vi "Load Hardware.vi"(8 "error in (no error)":errorcluster, 10 "Program only changes":bool=TRUE, 11 "ArduinoDAC in":refnum<class "ArduinoDAC.lvclass">) -> (0 "error out":errorcluster, 3 "ArduinoDAC out":refnum<class "ArduinoDAC.lvclass">)   [LabVIEW 2013, in "ArduinoDAC.lvclass"]
uses:
  ArduinoDAC.lvclass
  <vilib>/Instr/_visa.llb/VISA Open Access Mode.ctl
  ArduinoDAC.lvclass/ArduinoDAC.ctl
panel:
  # "encapsulate HWI in cluser so each \"last encountered\"\ncan be a different length."
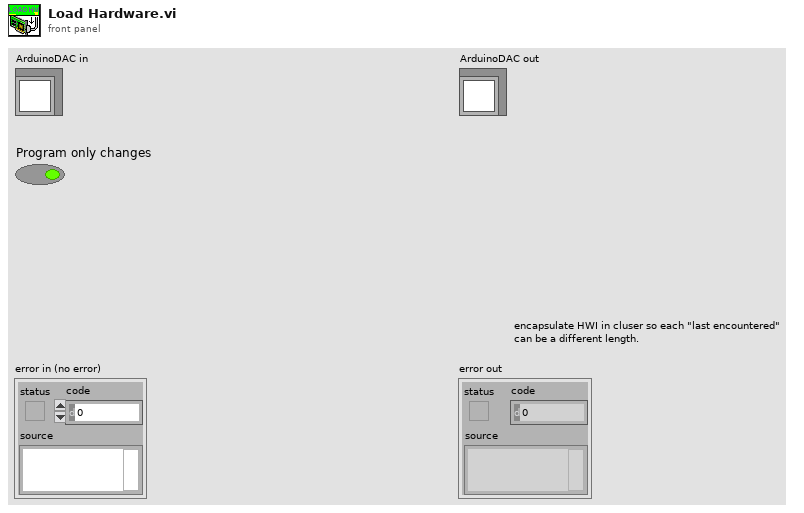
[diagram p1: front panel]
types:
  T1 = typedef "VISA Open Access Mode.ctl" = u32
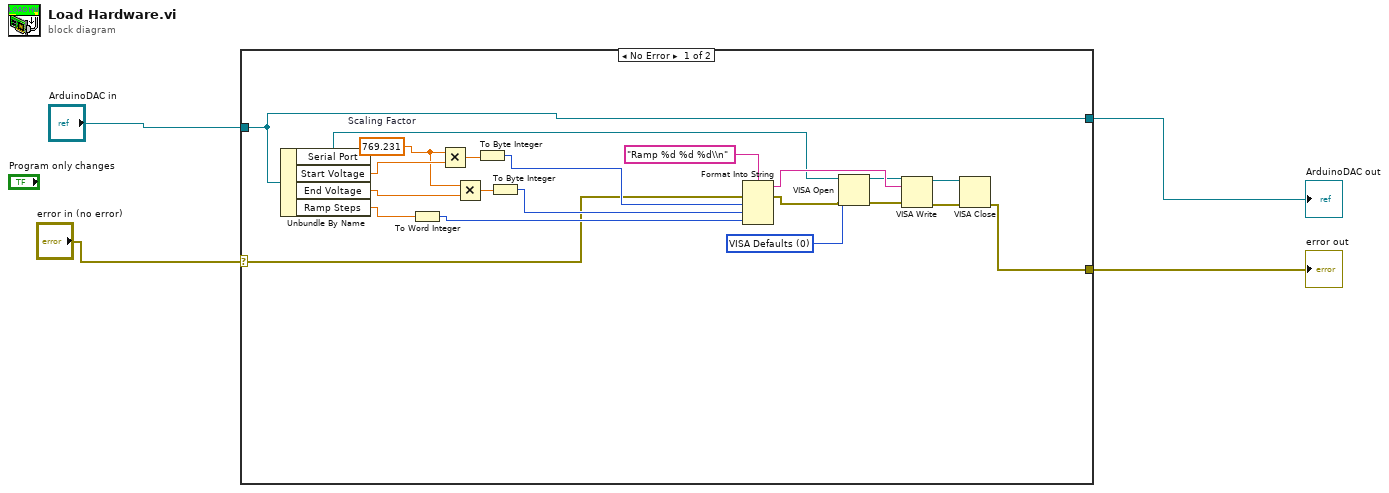
[diagram p0: block diagram]
diagram:
  n1 = case shown="No Error" "error in (no error)" {
    selector: "error in (no error)" -> [w14 w26]
    tunnel: "ArduinoDAC in" -> [w25 w27]
    tunnel: [w25 w27] -> w2
    tunnel: [w5 w26] -> w1
    frame No Error {
      w10 = T1 0 items=["VISA Defaults"=0, "Exclusive Lock"=1, "Load Configured Settings"=4] ("Access Mode")
      w23 = 769.231  # Scaling Factor
      n2 = Unbundle By Name(w25) -> ("Serial Port"=w12:refnum<visa-resource-name>, "Start Voltage"=w24:dbl, "End Voltage"=w22:dbl, "Ramp Steps"=w19:dbl)
      n3 = To Word Integer(number=w19) -> (16bit integer=w16:i16)
      n4 = Multiply(x=w23, y=w24) -> (x*y=w20:dbl)
      n5 = Multiply(x=w23, y=w22) -> (x*y=w21:dbl)
      n6 = To Byte Integer(number=w20) -> (8bit integer=w18:i8)
      n7 = To Byte Integer(number=w21) -> (8bit integer=w17:i8)
      n8 = Format Into String(format string="Ramp %d %d %d\\n", error in=w14, w18, w17, w16) -> (resulting string=w13:string, error out=w11:errorcluster)  [unwired: 1 in]
      n9 = VISA Open(access mode=w10, error in (no error)=w11, VISA resource name=w12) -> (VISA resource name=w9:refnum<visa-resource-name>, error out=w8:errorcluster)  [unwired: 2 in]
      n10 = VISA Write(VISA resource name=w9, write buffer=w13, error in (no error)=w8) -> (VISA resource name out=w7:refnum<visa-resource-name>, error out=w6:errorcluster)  [unwired: 1 out]
      n11 = VISA Close(VISA resource name=w7, error in (no error)=w6) -> (error out=w5:errorcluster)
    }
    frame Error {
    }
  }
  "error out" <- w1
  "ArduinoDAC out" <- w2
